vi "Get All Data.vi"(0 "Arduino Resource":T3, 5 "Device Address":T1 items=["0x68", "0x69"], 11 "error in (no error)":errorcluster) -> (4 "Arduino Resource":T3, 6 "Accel Data":T2, 8 "Temperature (°C)":dbl, 10 "Gyro Data":T2, 15 "error out":errorcluster)   [LabVIEW 2009, in "LIFA MPU-60X0.lvlib"]
uses:
  LIFA MPU-60X0.lvlib
  <vilib>/LabVIEW Interface for Arduino/LabVIEW Interface for Arduino.lvlib
  RegisterAddresses.ctl
  <vilib>/LabVIEW Interface for Arduino/Type Defs/Board Type.ctl
  <vilib>/LabVIEW Interface for Arduino/Type Defs/Arduino Resource.ctl
  DeviceAddresses.ctl
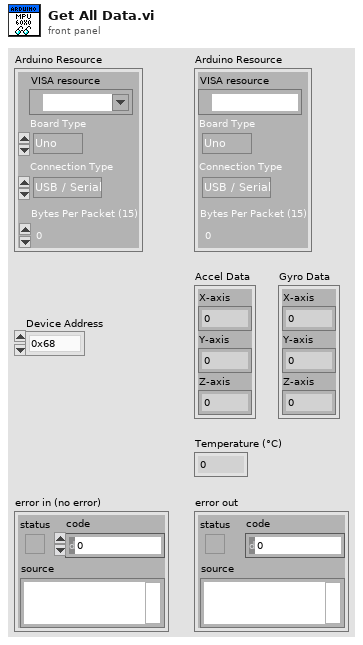
[diagram p1: front panel]
types:
  T1 = typedef "LIFA MPU-60X0.lvlib/DeviceAddresses.ctl" = u8
  T2 = cluster{"X-axis":i16, "Y-axis":i16, "Z-axis":i16}
  T3 = typedef "LabVIEW Interface for Arduino.lvlib/Arduino Resource.ctl" = cluster{"VISA resource":refnum<visa-resource-name>, "Board Type":T4, "Connection Type":enum8{"USB / Serial"}, "Bytes Per Packet (15)":u8}
  T4 = typedef "LabVIEW Interface for Arduino.lvlib/Board Type.ctl" = enum16{"Uno", "Dimuelanove w/Atmega 328", "Mega 2560"}
  T5 = typedef "LIFA MPU-60X0.lvlib/RegisterAddresses.ctl" = u16
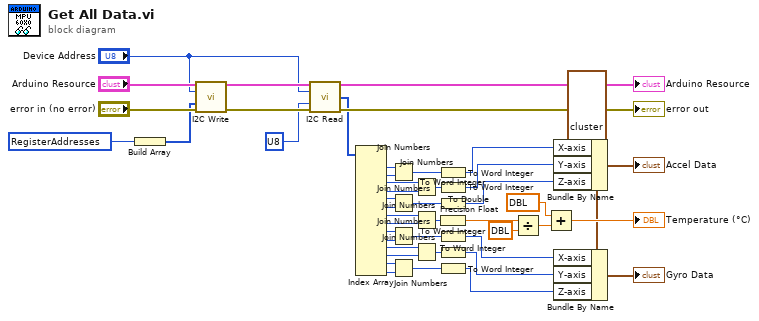
[diagram p0: block diagram]
diagram:
  w5 = T2 ? ("input cluster")
  w40 = T5 ? items=["SELF_TEST_X", "SELF_TEST_Y", "SELF_TEST_Z", "SELF_TEST_A", "SMPLRT_DIV", "CONFIG", "GYRO_CONFIG", "ACCEL_CONFIG", "MOT_THR", "FIFO_EN", "I2C_MST_CTRL", "I2C_SLV0_ADDR", "I2C_SLV0_REG", "I2C_SLV0_CTRL", "I2C_SLV1_ADDR", "I2C_SLV1_REG", "I2C_SLV1_CTRL", "I2C_SLV2_ADDR", "I2C_SLV2_REG", "I2C_SLV2_CTRL", "I2C_SLV3_ADDR", "I2C_SLV3_REG", "I2C_SLV3_CTRL", "I2C_SLV4_ADDR", "I2C_SLV4_REG", "I2C_SLV4_DO", "I2C_SLV4_CTRL", "I2C_SLV4_DI", "I2C_MST_STATUS", "INT_PIN_CFG", "INT_ENABLE", "INT_STATUS", "ACCEL_XOUT_H", "ACCEL_XOUT_L", "ACCEL_YOUT_H", "ACCEL_YOUT_L", "ACCEL_ZOUT_H", "ACCEL_ZOUT_L", "TEMP_OUT_H", "TEMP_OUT_L", "GYRO_XOUT_H", "GYRO_XOUT_L", "GYRO_YOUT_H", "GYRO_YOUT_L", "GYRO_ZOUT_H", "GYRO_ZOUT_L", "EXT_SENS_DATA_00", "EXT_SENS_DATA_01", "EXT_SENS_DATA_02", "EXT_SENS_DATA_03", "EXT_SENS_DATA_04", "EXT_SENS_DATA_05", "EXT_SENS_DATA_06", "EXT_SENS_DATA_07", "EXT_SENS_DATA_08", "EXT_SENS_DATA_09", "EXT_SENS_DATA_10", "EXT_SENS_DATA_11", "EXT_SENS_DATA_12", "EXT_SENS_DATA_13", "EXT_SENS_DATA_14", "EXT_SENS_DATA_15", "EXT_SENS_DATA_16", "EXT_SENS_DATA_17", "EXT_SENS_DATA_18", "EXT_SENS_DATA_19", "EXT_SENS_DATA_20", "EXT_SENS_DATA_21", "EXT_SENS_DATA_22", "EXT_SENS_DATA_23", "I2C_SLV0_DO", "I2C_SLV1_DO", "I2C_SLV2_DO", "I2C_SLV3_DO", "I2C_MST_DELAY_CTRL", "SIGNAL_PATH_RESET", "MOT_DETECT_CTRL", "USER_CTRL", "PWR_MGMT_1", "PWR_MGMT_2", "FIFO_COUNTH", "FIFO_COUNTL", "FIFO_R_W", "WHO_AM_I"] ("Register Addresses")
  n1 = Build Array(w40) -> (w39:T5[])
  n2 = call <vilib>:"I2C Write.vi"("Arduino Resource"="Arduino Resource", "Address (0)"="Device Address", "I2C Data Bytes"=w39, "error in"="error in (no error)") -> ("Arduino Resource"=w46:T3, "error out"=w45:errorcluster)  [unwired: 10 in]
  n3 = call <vilib>:"I2C Read.vi"("Arduino Resource"=w46, "Address (0)"="Device Address", "Bytes To Read"=u8 ?, "error in"=w45) -> ("Arduino Resource"=→"Arduino Resource":T3, "I2C Data"=w36:u8[], "error out"=→"error out":errorcluster)  [unwired: 9 in]
  n4 = Index Array(array=w36) -> (element #1=w35:u8, element #2=w34:u8, element #3=w33:u8, element #4=w32:u8, element #5=w31:u8, element #6=w30:u8, element #7=w29:u8, element #8=w28:u8, element #9=w27:u8, element #10=w26:u8, element #11=w25:u8, element #12=w24:u8, element #13=w23:u8, element #14=w22:u8)  [unwired: 14 in]
  n5 = Join Numbers(hi=w35, lo=w34) -> ((hi.lo)=w20:u16)
  n6 = Join Numbers(hi=w31, lo=w30) -> ((hi.lo)=w19:u16)
  n7 = Join Numbers(hi=w27, lo=w26) -> ((hi.lo)=w15:u16)
  n8 = Join Numbers(hi=w23, lo=w22) -> ((hi.lo)=w16:u16)
  n9 = Join Numbers(hi=w33, lo=w32) -> ((hi.lo)=w21:u16)
  n10 = Join Numbers(hi=w29, lo=w28) -> ((hi.lo)=w18:u16)
  n11 = Join Numbers(hi=w25, lo=w24) -> ((hi.lo)=w17:u16)
  n12 = To Word Integer(number=w20) -> (16bit integer=w9:i16)
  n13 = To Word Integer(number=w21) -> (16bit integer=w8:i16)
  n14 = To Word Integer(number=w19) -> (16bit integer=w7:i16)
  n15 = To Double Precision Float(number=w18) -> (double precision float=w14:dbl)
  n16 = To Word Integer(number=w15) -> (16bit integer=w4:i16)
  n17 = To Word Integer(number=w17) -> (16bit integer=w3:i16)
  n18 = To Word Integer(number=w16) -> (16bit integer=w2:i16)
  n19 = Divide(x=w14, y=dbl ?) -> (x/y=w12:dbl)
  n20 = Add(x=dbl ?, y=w12) -> (x+y=→"Temperature (°C)":dbl)
  n21 = Bundle By Name(cluster=w5, "X-axis"=w9, "Y-axis"=w8, "Z-axis"=w7) -> (→"Accel Data":T2)
  n22 = Bundle By Name(cluster=w5, "X-axis"=w4, "Y-axis"=w3, "Z-axis"=w2) -> (→"Gyro Data":T2)
